vi "ROI_coord2array.vi"(11 "Array in":i32[](array[numeric])) -> (3 "array out":i32[][](array[numeric]))   [LabVIEW 2017]
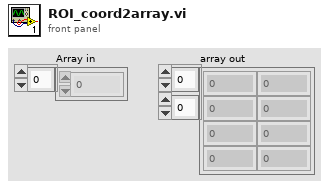
[diagram p1: front panel]
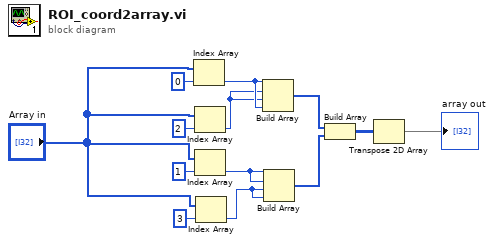
[diagram p0: block diagram]
diagram:
  n1 = Index Array(array="Array in", index=0) -> (element=w13:i32)
  n2 = Index Array(array="Array in", index=2) -> (element=w12:i32)
  n3 = Index Array(array="Array in", index=1) -> (element=w6:i32)
  n4 = Index Array(array="Array in", index=3) -> (element=w7:i32)
  n5 = Build Array(w13, w12, w12, w13) -> (w8:i32[])
  n6 = Build Array(w6, w6, w7, w7) -> (w9:i32[])
  n7 = Build Array(w8, w9) -> (w10:i32[][])
  n8 = Transpose 2D Array(2D array=w10) -> (transposed array=→"array out":i32[][])
